vi "Wave Graph vs Chart.vi"() -> ()   [LabVIEW 2023]
panel:
  out "Array":dbl[](array[numeric]) format="%#_2g"
  out "XY Graph":cluster{dbl[], dbl[]}(graph)
  out "Waveform Graph 2":dbl[](graph)
  out "Waveform Graph":dbl[][](graph)
  out "Waveform Chart":dbl(graph)
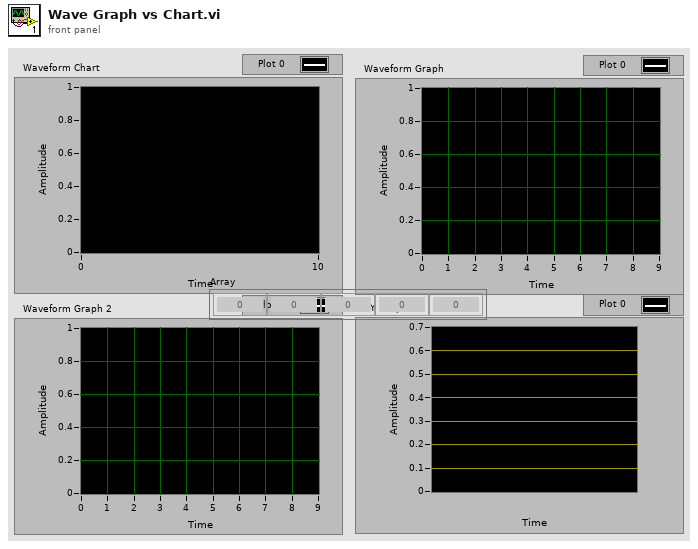
[diagram p1: front panel]
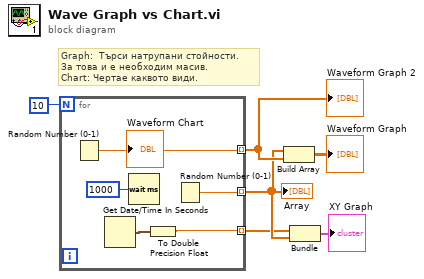
[diagram p0: block diagram]
diagram:
  # "Graph:  Търси натрупани стойности.\nЗа това и е необходим масив.\nChart: Чертае каквото види."
  n1 = for {
    N: 10 -> [_]
    tunnel: [w11] -> w4 mode=indexing
    tunnel: [w10] -> w2 mode=indexing
    tunnel: [w8] -> w1 mode=indexing
    n2 = Random Number (0-1)() -> (number: 0 to 1=w11:dbl)
    "Waveform Chart" <- w11
    n3 = Get Date/Time In Seconds() -> (seconds since 1Jan1904=w9:timestamp)
    n4 = Wait (ms)(milliseconds to wait=u32 1000) -> ()  [unwired: 1 out]
    n5 = To Double Precision Float(number=w9) -> (double precision float=w8:dbl)
    n6 = Random Number (0-1)() -> (number: 0 to 1=w10:dbl)
  }
  "Waveform Graph 2" <- w4
  "Array" <- w2
  n7 = Build Array(w2, w4) -> (→"Waveform Graph":dbl[][])
  n8 = Bundle(w1, w2) -> (→"XY Graph":cluster{dbl[], dbl[]})  [unwired: 1 in]
